vi "Monitoring task.vi"   [LabVIEW 2016]
types:
  T1 = enum16{"启动测量", "标样核查", "零点核查", "跨度核查", "空白测试", "平行样测试", "加标回收", "空白校准", "标样校准", "初始化（清洗）", "停止测试", "仪器重启", "校时", "模式设置", "测量间隔设置"}
  T2 = cluster{"测试模式":enum16{"水样测试", "平行样测试", "集成干预测试", "加标回收"}, "参数启用":cluster{"多参数":bool, "湿化学":bool}}
  T3 = typedef "控制命令与参数.ctl" = cluster{"控制命令":enum16{"启动测量", "标样核查", "零点核查", "跨度核查", "空白测试", "平行样测试", "加标回收", "空白校准", "标样校准", "初始化（清洗）", "停止测试", "仪器重启", "校时", "模式设置", "测量间隔设置"}, "测量参数":string}
  T4 = typedef "斯坦道原位多参数.lvlib/水样测试启动自定义输入参数.ctl" = cluster{"测量模式":string, "数据类型":string}
  T5 = cluster{"运行模式":enum16{"维护模式", "常规模式", "应急模式", "质控模式"}, "质控频次":enum16{"关闭", "每天", "星期一", "星期二", "星期三", "星期四", "星期五", "星期六", "星期日"}, "空白核查时间":u16, "跨度核查时间":u16, "多参数测试间隔":u16, "湿化学测试间隔":u16}
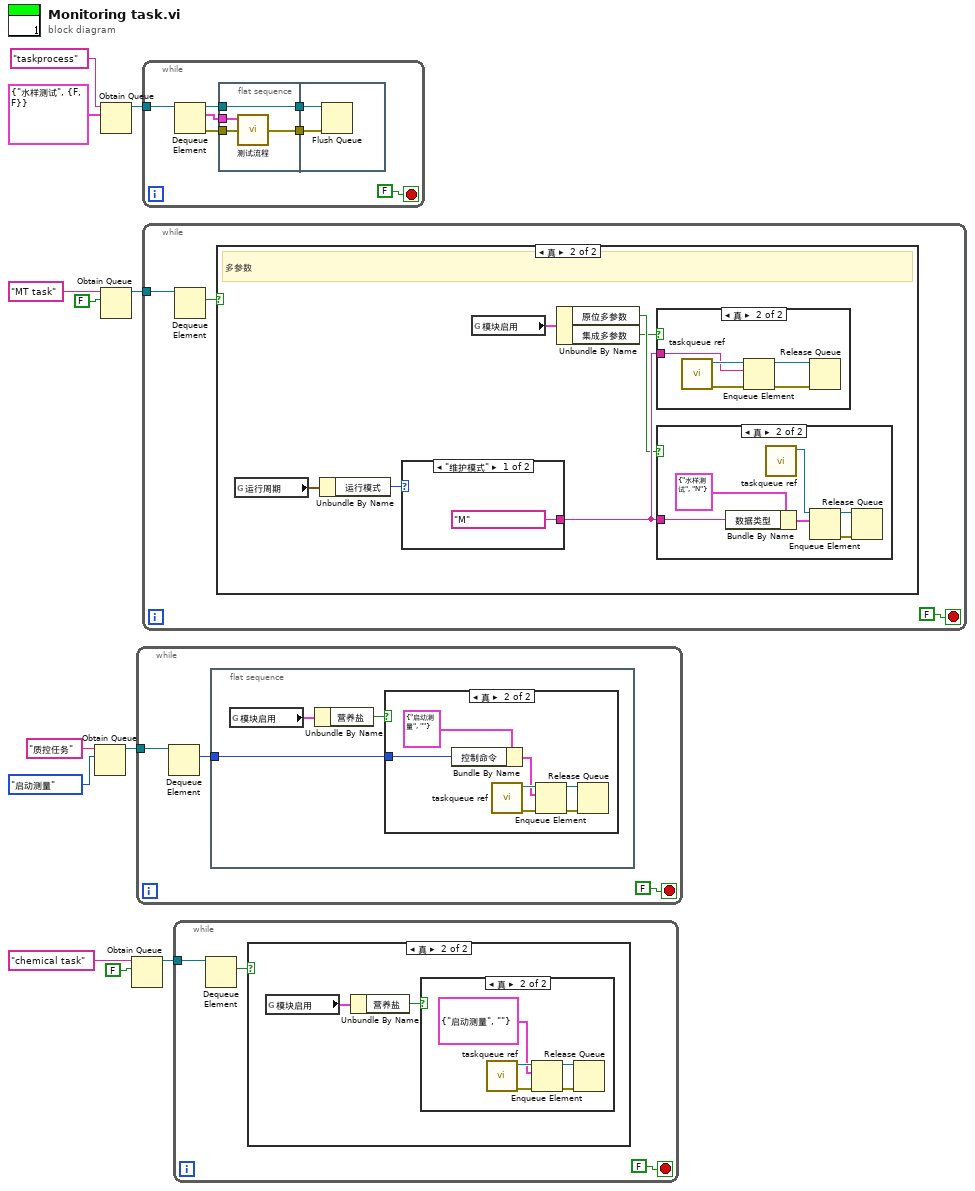
[diagram p0: block diagram]
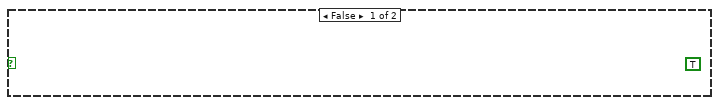
[diagram p5: hidden frame]
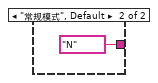
[diagram p8: hidden frame]
diagram:
  n1 = Obtain Queue(name (unnamed)="质控任务" ("名称（未命名）"), element data type=T1."启动测量" ("控制命令")) -> (queue out=w4:refnum<queue>)  [unwired: 3 in, 2 out]
  n2 = Obtain Queue(name (unnamed)="taskprocess" ("名称（未命名）"), element data type=T2 {"测试模式"=enum."水样测试", "参数启用"={"多参数"=FALSE, "湿化学"=FALSE}} ("参数")) -> (queue out=w8:refnum<queue>)  [unwired: 3 in, 2 out]
  n3 = Obtain Queue(name (unnamed)="MT task" ("名称（未命名）"), element data type=FALSE) -> (queue out=w11:refnum<queue>)  [unwired: 3 in, 2 out]
  n4 = Obtain Queue(name (unnamed)="chemical task" ("名称（未命名）"), element data type=FALSE) -> (queue out=w3:refnum<queue>)  [unwired: 3 in, 2 out]
  n5 = while {
    tunnel: w4 -> [w14]
    stop <- FALSE stop-if-true
    n6 = Dequeue Element(queue=w14) -> (element=w13:T1)  [unwired: 2 in, 3 out]
    n7 = flat-sequence {
      tunnel: w13 -> [w18]
      frame #0 {
        n8 = global read "系统设置全局变量.vi" "模块启用"() -> (w17:cluster{"原位多参数":bool, "集成多参数":bool, "营养盐":bool})
        n9 = Unbundle By Name(w17) -> ("营养盐"=w16:bool)
        n10 = case shown="真" w16 {
          tunnel: w18 -> [_ w19]
          frame False {
          }
          frame True {
            n11 = Bundle By Name(cluster=T3 {"控制命令"=enum."启动测量", "测量参数"=""} ("元素"), "控制命令"=w19) -> (w20:T3)
            n12 = call "taskqueue ref.vi"() -> ("错误输出"=w22:errorcluster, "队列输出"=w23:refnum<queue>)  [unwired: 10 in]
            n13 = Enqueue Element(queue=w23, element=w20, error in (no error)=w22) -> (queue out=w25:refnum<queue>, error out=w24:errorcluster)  [unwired: 1 in, 1 out]
            n14 = Release Queue(queue=w25, error in (no error)=w24) -> ()  [unwired: 1 in, 3 out]
          }
        }
      }
    }
  }
  n15 = while {
    tunnel: w8 -> [w32]
    stop <- FALSE stop-if-true
    n16 = Dequeue Element(queue=w32) -> (queue out=w29:refnum<queue>, element=w30:T2, error out=w26:errorcluster)  [unwired: 2 in, 1 out]
    n17 = flat-sequence {
      tunnel: w30 -> [w35]
      tunnel: w29 -> [w34]
      tunnel: [w34] -> w28
      tunnel: [w33] -> w27
      tunnel: w26 -> [w33]
      tunnel: w28 -> [w37]
      tunnel: w27 -> [w36]
      frame #0 {
        n18 = call "测试流程.vi"("参数"=w35) -> ()  [unwired: 11 in]
      }
      frame #1 {
        n19 = Flush Queue(queue=w37, error in (no error)=w36) -> ()  [unwired: 3 out]
      }
    }
  }
  n20 = while {
    tunnel: w11 -> [w40]
    stop <- FALSE stop-if-true
    n21 = Dequeue Element(queue=w40) -> (element=w39:bool)  [unwired: 2 in, 3 out]
    n22 = case shown="真" w39 {
      frame False {
        (unwired) TRUE ("t")
      }
      frame True {
        # "多参数"
        n23 = global read "系统设置全局变量.vi" "运行周期"() -> (w46:T5)
        n24 = Unbundle By Name(w46) -> ("运行模式"=w45:enum16{"维护模式", "常规模式", "应急模式", "质控模式"})
        n25 = case shown="\"维护模式\"" w45 {
          tunnel: ["M" ("数据标记表") "N" ("数据标记表")] -> w44
          frame "维护模式" {
          }
          frame "常规模式", Default {
          }
        }
        n26 = global read "系统设置全局变量.vi" "模块启用"() -> (w43:cluster{"原位多参数":bool, "集成多参数":bool, "营养盐":bool})
        n27 = Unbundle By Name(w43) -> ("原位多参数"=w42:bool, "集成多参数"=w41:bool)
        n28 = case shown="真" w41 {
          tunnel: w44 -> [_ w47]
          frame False {
          }
          frame True {
            n29 = call "taskqueue ref.vi"() -> ("错误输出"=w49:errorcluster, "队列输出"=w48:refnum<queue>)  [unwired: 10 in]
            n30 = Enqueue Element(queue=w48, element=w47, error in (no error)=w49) -> (queue out=w50:refnum<queue>, error out=w51:errorcluster)  [unwired: 1 in, 1 out]
            n31 = Release Queue(queue=w50, error in (no error)=w51) -> ()  [unwired: 1 in, 3 out]
          }
        }
        n32 = case shown="真" w42 {
          tunnel: w44 -> [_ w52]
          frame False {
          }
          frame True {
            n33 = Bundle By Name(cluster=T4 {"测量模式"="水样测试", "数据类型"="N"} ("元素"), "数据类型"=w52) -> (w53:T4)
            n34 = call "taskqueue ref.vi"() -> ("队列输出"=w55:refnum<queue>)  [unwired: 10 in, 1 out]
            n35 = Enqueue Element(queue=w55, element=w53) -> (queue out=w57:refnum<queue>, error out=w56:errorcluster)  [unwired: 2 in, 1 out]
            n36 = Release Queue(queue=w57, error in (no error)=w56) -> ()  [unwired: 1 in, 3 out]
          }
        }
      }
    }
  }
  n37 = while {
    tunnel: w3 -> [w61]
    stop <- FALSE stop-if-true
    n38 = Dequeue Element(queue=w61) -> (element=w60:bool)  [unwired: 2 in, 3 out]
    n39 = case shown="真" w60 {
      frame False {
      }
      frame True {
        n40 = global read "系统设置全局变量.vi" "模块启用"() -> (w64:cluster{"原位多参数":bool, "集成多参数":bool, "营养盐":bool})
        n41 = Unbundle By Name(w64) -> ("营养盐"=w63:bool)
        n42 = case shown="真" w63 {
          frame False {
          }
          frame True {
            n43 = call "taskqueue ref.vi"() -> ("错误输出"=w68:errorcluster, "队列输出"=w69:refnum<queue>)  [unwired: 10 in]
            n44 = Enqueue Element(queue=w69, element=T3 {"控制命令"=enum."启动测量", "测量参数"=""} ("元素"), error in (no error)=w68) -> (queue out=w67:refnum<queue>, error out=w66:errorcluster)  [unwired: 1 in, 1 out]
            n45 = Release Queue(queue=w67, error in (no error)=w66) -> ()  [unwired: 1 in, 3 out]
          }
        }
      }
    }
  }
